vi "Disk Information.vi"(7 "path":path=path "D:/") -> (0 "free (Gb)":dbl format="%.2f", 1 "size (Gb)":dbl format="%.2f", 2 "Option":T1, 3 "Harddisk size":dbl(slide) caption="6.06 %" scale=0.0..100.0)   [LabVIEW 2017]
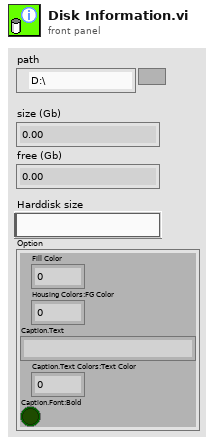
[diagram p1: front panel]
types:
  T1 = cluster{"Fill Color":u32, "Housing Colors:FG Color":u32, "Caption.Text":string, "Caption.Text Colors:Text Color":u32, "Caption.Font:Bold":bool}
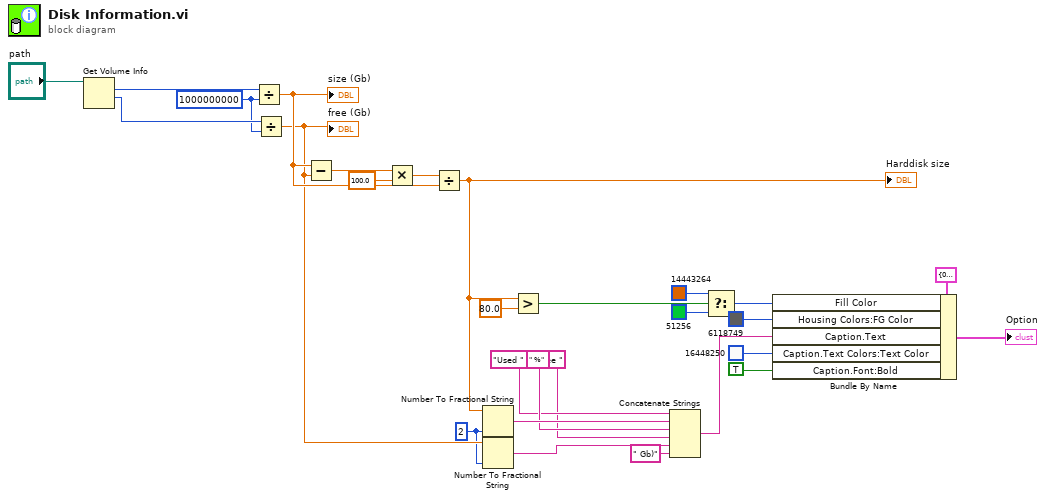
[diagram p0: block diagram]
diagram:
  w3 = i16 2 ("precision (6)")
  w14 = i64 1000000000 ("y")
  n1 = Get Volume Info(11:"path") -> (1:w26:i64, 2:w27:i64)  [unwired: 1 in, 4 out]
  n2 = Divide(x=w27, y=w14) -> (x/y=w23:dbl)
  "size (Gb)" <- w23
  n3 = Divide(x=w26, y=w14) -> (x/y=w4:dbl)
  "free (Gb)" <- w4
  n4 = Subtract(x=w23, y=w4) -> (x-y=w22:dbl)
  n5 = Multiply(x=w22, y=100.0) -> (x*y=w24:dbl)
  n6 = Divide(x=w24, y=w23) -> (x/y=w19:dbl)
  "Harddisk size" <- w19
  n7 = Number To Fractional String(number=w19, precision (6)=w3) -> (F-format string=w21:string)  [unwired: 2 in]
  n8 = Number To Fractional String(number=w4, precision (6)=w3) -> (F-format string=w2:string)  [unwired: 2 in]
  n9 = Greater?(x=w19, y=80.0) -> (0:w17:bool)
  n10 = Concatenate Strings("Used " ("string"), w21, " %" ("string"), " (Free " ("string"), w2, " Gb)" ("string")) -> (w10:string)
  n11 = Select(t=u32 14443264, s=w17, f=u32 51256) -> (s? t:f=w12:u32)
  n12 = Bundle By Name(cluster=T1 {"Fill Color"=0, "Housing Colors:FG Color"=0, "Caption.Text"="", "Caption.Text Colors:Text Color"=0, "Caption.Font:Bold"=FALSE}, "Fill Color"=w12, "Housing Colors:FG Color"=u32 6118749, "Caption.Text"=w10, "Caption.Text Colors:Text Color"=u32 16448250, "Caption.Font:Bold"=TRUE) -> (→"Option":T1)
